vi "Prober_ReadXYZTheta.vi"(8 "error in (no error)":errorcluster, 11 "AlessiRel6100 in":refnum<class "AlessiRel6100.lvclass">) -> (0 "error out":errorcluster, 1 "Z location [µm]":i32, 2 "Y location [µm]":i32, 3 "X location [µm]":i32, 4 "Theta location [mdeg]":i32, 5 "AlessiRel6100 out":refnum<class "AlessiRel6100.lvclass">)   [LabVIEW 2013, in "AlessiRel6100.lvclass"]
uses:
  AlessiRel6100.lvclass
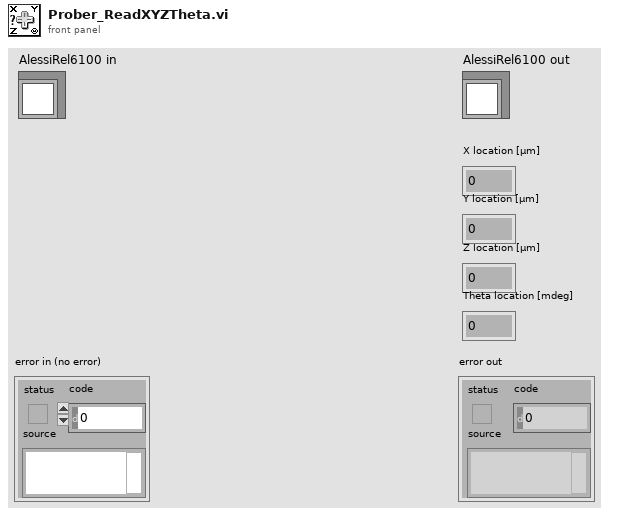
[diagram p1: front panel]
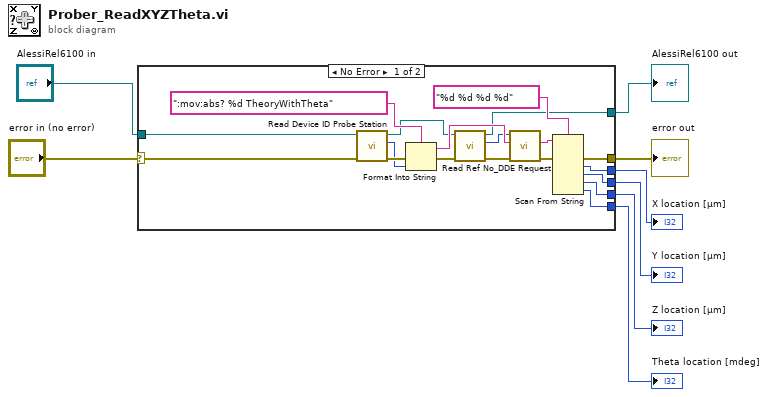
[diagram p0: block diagram]
diagram:
  n1 = case shown="No Error" "error in (no error)" {
    selector: "error in (no error)" -> [w17 w29]
    tunnel: [w23 w29] -> w5
    tunnel: "AlessiRel6100 in" -> [w18 w28]
    tunnel: [w22 _] -> w4
    tunnel: [w21 _] -> w3
    tunnel: [w20 _] -> w2
    tunnel: [w19 _] -> w1
    tunnel: [w9 w28] -> w6
    frame No Error {
      n2 = call-dynamic "Read Device ID Probe Station.vi"("error in (no error)"=w17, "AlessiRel6100 in"=w18) -> ("error out"=w15:errorcluster, "Device ID Probe Station"=w10:u32, "AlessiRel6100 out"=w16:refnum<class "AlessiRel6100.lvclass">)  [unwired: 7 in]
      n3 = Format Into String(format string=":mov:abs? %d TheoryWithTheta", error in=w15, w10) -> (resulting string=w27:string, error out=w14:errorcluster)  [unwired: 1 in]
      n4 = call-dynamic "Read Ref No_.vi"("error in (no error)"=w14, "AlessiRel6100 in"=w16) -> ("error out"=w13:errorcluster, "Ref No."=w12:u32, "AlessiRel6100 out"=w9:refnum<class "AlessiRel6100.lvclass">)  [unwired: 7 in]
      n5 = call <vilib>:"DDE Request.vi"("error in (no error)"=w13, "item"=w27, "conversation refnum in"=w12) -> ("error out"=w25:errorcluster, "data"=w11:string)  [unwired: 4 in, 1 out]
      n6 = Scan From String(format string="%d %d %d %d", input string=w11, error in=w25) -> (error out=w23:errorcluster, output 1=w22:i32, output 2=w21:i32, output 3=w20:i32, output 4=w19:i32)  [unwired: 5 in, 2 out]
    }
    frame Error {
    }
  }
  "error out" <- w5
  "X location [µm]" <- w4
  "Z location [µm]" <- w2
  "Theta location [mdeg]" <- w1
  "Y location [µm]" <- w3
  "AlessiRel6100 out" <- w6
